vi "using_arrays_and_loops.vi"() -> ()   [LabVIEW 2023]
panel:
  in  "stop 2":bool
  out "dongu":i32
  out "kayıt verisi":string
  out "Array 3":dbl[](array[numeric])
  out "min value":dbl
  out "max value":dbl
  out "while dongusu":dbl[](array[numeric])
  in  "stop":bool
  out "for dongusu":dbl[](array[numeric])
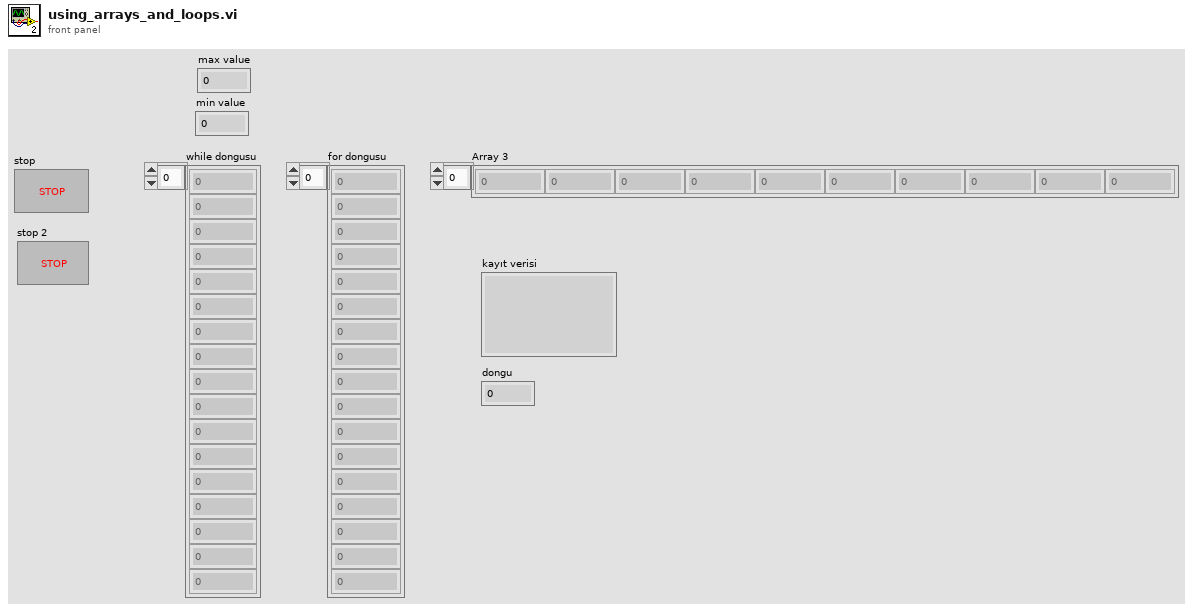
[diagram p1: front panel]
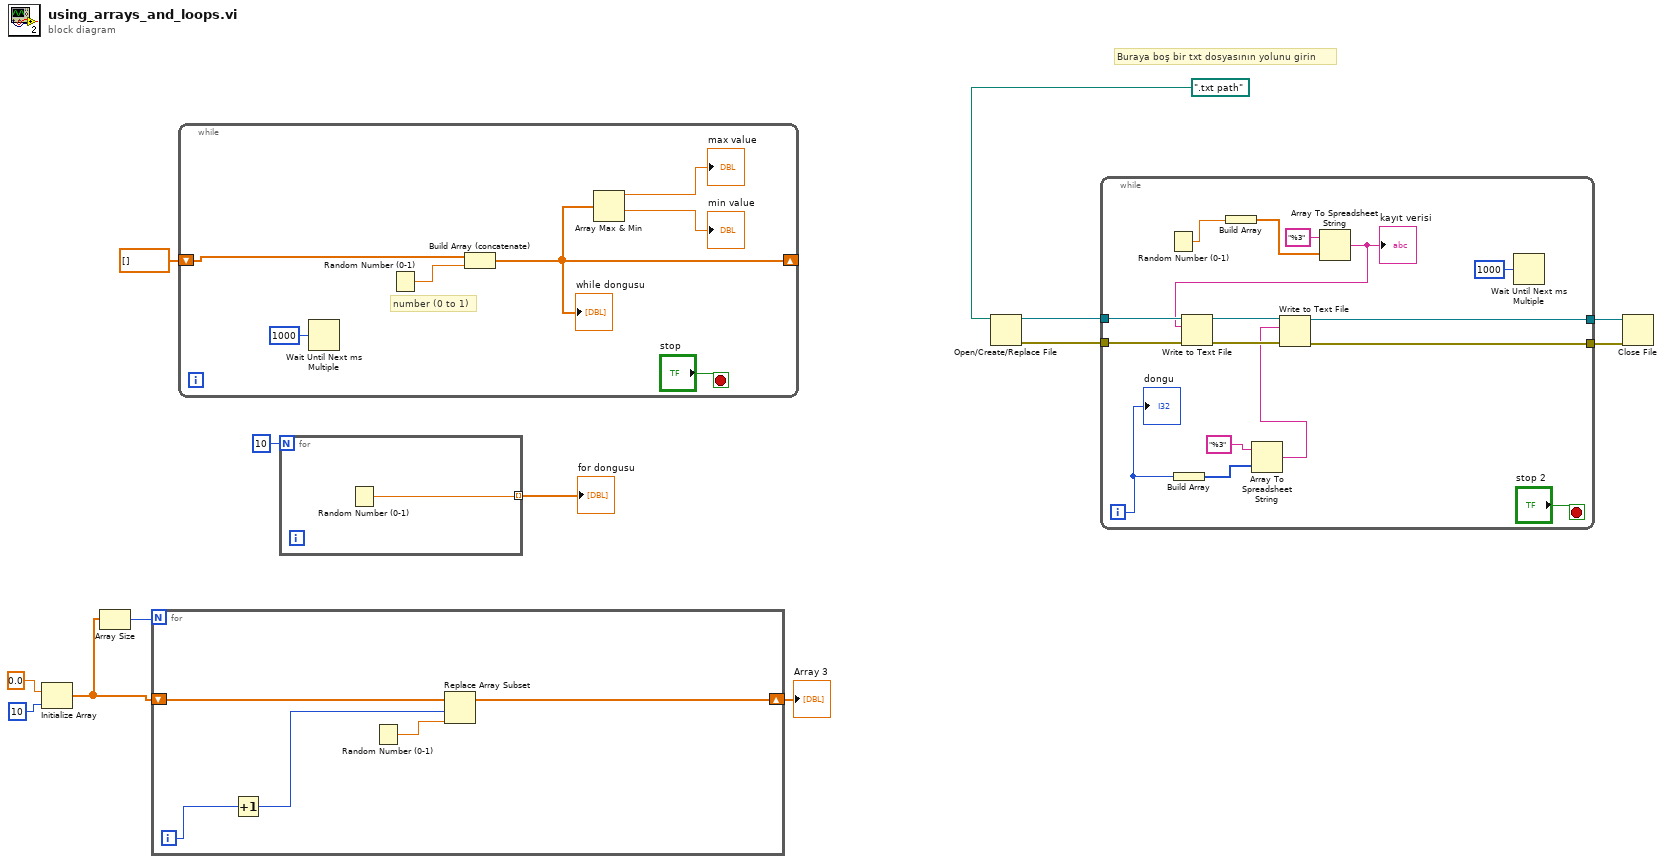
[diagram p0: block diagram]
diagram:
  # "Buraya boş bir txt dosyasının yolunu girin"
  n1 = Initialize Array(0.0 ("element"), 10 ("dimension size")) -> (w7:dbl[])
  n2 = Array Size(array=w7) -> (size(s)=w8:i32)
  n3 = for {
    N: w8 -> [_]
    shift-right: [w15] -> w6
    shift-left: w7 -> [w14]
    i -> [w18]
    n4 = Increment(x=w18) -> (x+1=w16:i32)
    n5 = Random Number (0-1)() -> (number: 0 to 1=w17:dbl)
    n6 = Replace Array Subset(array=w14, new element=w17, index=w16) -> (w15:dbl[])
  }
  "Array 3" <- w6
  n7 = while {
    shift-right: [w21] -> _
    shift-left: dbl[] [] -> [w22]
    stop <- "stop" stop-if-true
    # "number (0 to 1)"
    n8 = Wait Until Next ms Multiple(millisecond multiple=u32 1000) -> ()  [unwired: 1 out]
    n9 = Random Number (0-1)() -> (number: 0 to 1=w24:dbl)
    n10 = Build Array (concatenate)(w22, w24) -> (w21:dbl[])
    "while dongusu" <- w21
    n11 = Array Max & Min(array=w21) -> (max value=→"max value":dbl, min value=→"min value":dbl)  [unwired: 2 out]
  }
  n12 = for {
    N: 10 -> [_]
    tunnel: [w26] -> w12 mode=indexing
    n13 = Random Number (0-1)() -> (number: 0 to 1=w26:dbl)
  }
  "for dongusu" <- w12
  n14 = Open/Create/Replace File(file path (use dialog)=path ".txt path") -> (refnum out=w4:refnum<file>, error out=w3:errorcluster)  [unwired: 5 in, 1 out]
  n15 = while {
    tunnel: w4 -> [w38]
    tunnel: w3 -> [w37]
    tunnel: [w28] -> w2
    tunnel: [w27] -> w1
    i -> [w35]
    stop <- "stop 2" stop-if-true
    n16 = Random Number (0-1)() -> (number: 0 to 1=w41:dbl)
    n17 = Build Array(w35) -> (w32:i32[])
    n18 = Build Array(w41) -> (w40:dbl[])
    n19 = Array To Spreadsheet String(array=w32, 3:"%3" ("format string")) -> (spreadsheet string=w30:string)  [unwired: 1 in]
    n20 = Array To Spreadsheet String(array=w40, 3:"%3" ("format string")) -> (spreadsheet string=w36:string)  [unwired: 1 in]
    "kayıt verisi" <- w36
    n21 = Write to Text File(file (use dialog)=w38, text=w36, error in=w37) -> (refnum out=w34:refnum<file>, error out=w33:errorcluster)  [unwired: 1 in, 1 out]
    n22 = Write to Text File(file (use dialog)=w34, text=w30, error in=w33) -> (refnum out=w28:refnum<file>, error out=w27:errorcluster)  [unwired: 1 in, 1 out]
    n23 = Wait Until Next ms Multiple(millisecond multiple=u32 1000) -> ()  [unwired: 1 out]
    "dongu" <- w35
  }
  n24 = Close File(refnum=w2, error in=w1) -> ()  [unwired: 2 out]
